vi "SubPanel.vi"(0 "Ref In":refnum<vi>[](array[refnum]), 5 "VI reference":refnum<vi>, 11 "error in (no error)":errorcluster) -> (4 "Ref Out":refnum<vi>[](array[refnum]), 15 "error out":errorcluster)   [LabVIEW 2015, in "Drona basic.lvlib"]
doc: "This VI gets the references of all the controls present in the subpanel"
uses:
  Drona basic.lvlib
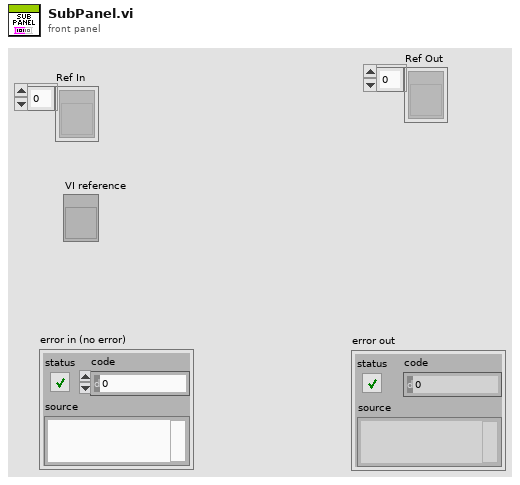
[diagram p1: front panel]
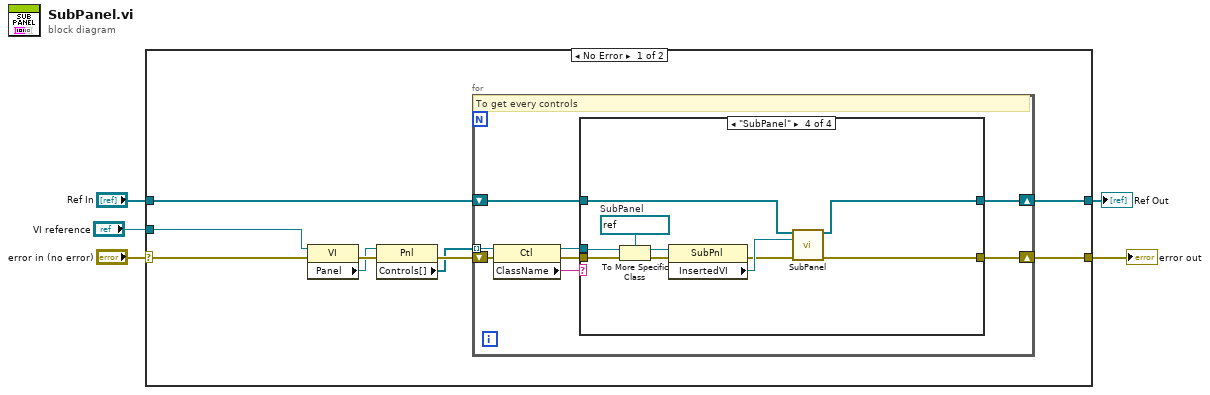
[diagram p0: block diagram]
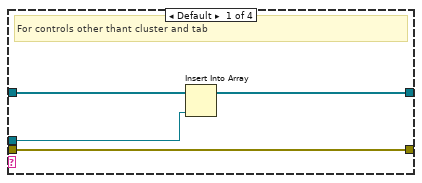
[diagram p2: hidden frame]
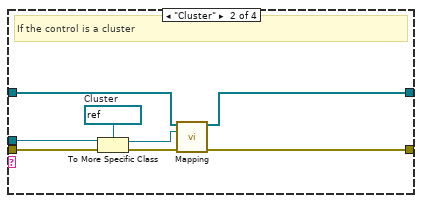
[diagram p3: hidden frame]
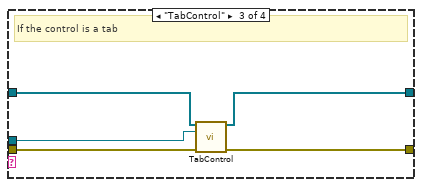
[diagram p4: hidden frame]
diagram:
  n1 = case shown="No Error" "error in (no error)" {
    selector: "error in (no error)" -> [w10 w51]
    tunnel: [w9 w50] -> w3
    tunnel: [w8 w51] -> w4
    tunnel: "Ref In" -> [w7 w50]
    tunnel: "VI reference" -> [w6 _]
    frame No Error {
      n2 = property class="VI"(reference=w6, error in=w10) -> (error out=w14:errorcluster, "Panel"=w13:refnum<vi>)  [unwired: 1 out]
      n3 = property class="Pnl"(reference=w13, error in=w14) -> (error out=w12:errorcluster, "Controls[]"=w11:refnum<vi>[])  [unwired: 1 out]
      n4 = for {
        shift-right: [w22] -> w8
        shift-left: w12 -> [w21]
        tunnel: w11 -> [w19] mode=indexing
        shift-right: [w15] -> w9
        shift-left: w7 -> [w17]
        # "To get every controls"
        n5 = property class="Ctl"(reference=w19, error in=w21) -> (reference out=w16:refnum<vi>, error out=w20:errorcluster, "ClassName"=w18:string)
        n6 = case shown="\"SubPanel\"" w18 {
          tunnel: [w26 w34 w39 w42] -> w22
          tunnel: w20 -> [w26 w29 w38 w49]
          tunnel: w17 -> [w25 w33 w36 w40]
          tunnel: w16 -> [w23 w31 w37 w47]
          tunnel: [w24 w27 w35 w41] -> w15
          frame Default {
            # "For controls other thant cluster and tab"
            n7 = Insert Into Array(array=w25, new element=w23) -> (w24:refnum<vi>[])  [unwired: 1 in]
          }
          frame "Cluster" {
            w28 = refnum<vi> refnum  # Cluster
            # "If the control is a cluster"
            n8 = To More Specific Class(target class=w28, reference=w31, error in=w29) -> (specific class reference=w32:refnum<vi>, error out=w30:errorcluster)
            n9 = call "Mapping.vi"("Ref In"=w33, "Clust Refnum"=w32, "error in (no error)"=w30) -> ("Ref Out"=w27:refnum<vi>[], "error out"=w34:errorcluster)  [unwired: 11 in]
          }
          frame "TabControl" {
            # "If the control is a tab"
            n10 = call "TabControl.vi"("Ref In"=w36, "Ctl Refnum"=w37, "error in (no error)"=w38) -> ("Ref Out"=w35:refnum<vi>[], "error out"=w39:errorcluster)  [unwired: 11 in]
          }
          frame "SubPanel" {
            w46 = refnum<vi> refnum  # SubPanel
            n11 = To More Specific Class(target class=w46, reference=w47, error in=w49) -> (specific class reference=w45:refnum<vi>, error out=w48:errorcluster)
            n12 = property class="SubPnl"(reference=w45, error in=w48) -> (error out=w43:errorcluster, "InsertedVI"=w44:refnum<vi>)  [unwired: 1 out]
            n13 = call "SubPanel.vi"("Ref In"=w40, "VI reference"=w44, "error in (no error)"=w43) -> ("Ref Out"=w41:refnum<vi>[], "error out"=w42:errorcluster)  [unwired: 11 in]
          }
        }
      }
    }
    frame Error {
    }
  }
  "error out" <- w4
  "Ref Out" <- w3
